vi "Read tag select.vi"(8 "error in (no error)":errorcluster, 11 "alarms module configuration in":refnum<class "tag select module configuration.lvclass">) -> (0 "error out":errorcluster, 2 "alarms":T1[](array[typedef]), 3 "alarms module configuration out":refnum<class "tag select module configuration.lvclass">)   [LabVIEW 2013, in "tag select module configuration.lvclass"]
uses:
  tag select module configuration.lvclass
  tag select configuration.ctl
  <vilib>/NI/Tag Bus Module Framework/channel/TBM channel.lvclass
  tag select module configuration.lvclass/tag select module configuration.ctl
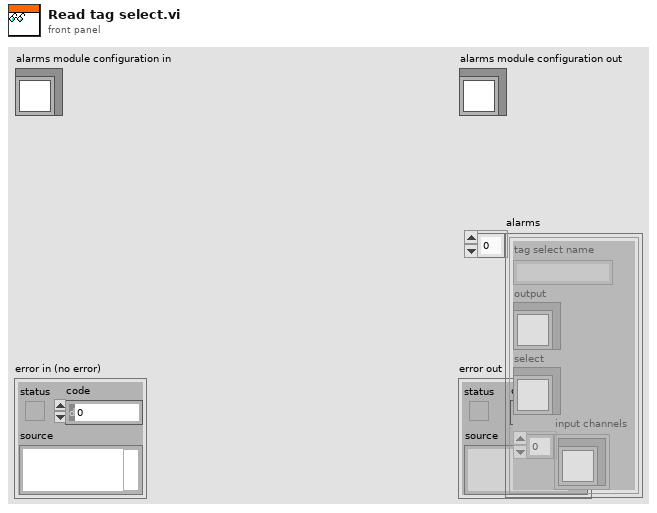
[diagram p1: front panel]
types:
  T1 = typedef "tag select module configuration.lvclass/tag select configuration.ctl" = cluster{"tag select name":string, "output":refnum<class "TBM channel.lvclass">, "select":refnum<class "TBM channel.lvclass">, "input channels":refnum<class "TBM channel.lvclass">[]}
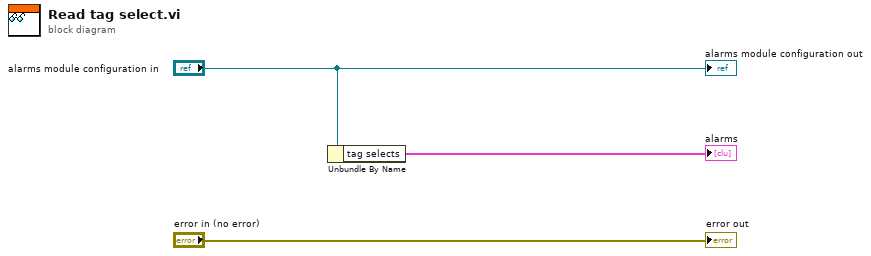
[diagram p0: block diagram]
diagram:
  n1 = Unbundle By Name("alarms module configuration in") -> ("tag selects"=→"alarms":T1[])
  "error out" <- "error in (no error)"
  "alarms module configuration out" <- "alarms module configuration in"
